vi "RT Main_V2 config.vi"   [LabVIEW 2015]
doc: "This template is for the Queued Message Handler design pattern.\n\nThe Event Handling Loop generates messages based on user interface actions.\n\nThe Message Handling Loop processes messages generated by the Event Handling Loop, or by other messages. The messages are string values, so new messages can be added easily to the Message Cases case structure in the Message Handling Loop. Each message cluster can also provide an optional value for Message Data, which is a variant that can be converted to whatever message-specific data is required."
uses:
  Globals/Global - All RT Loop Stop.vi
  Globals/Global - Monitoring Variables.vi
  Globals/Global - Configuration Options.vi
  Globals/Global - RT Stream Connections.vi
  support/Message Queue/Message Queue.lvlib
  <vilib>/nisyscfg/nisyscfg.lvlib
types:
  T1 = typedef "Acquisition and Logging Configuration_v1.ctl" = cluster{"Data Rate":T2, "Samples per Read":i32, "Number of Reads to Save":i32, "Data File Name":string, "TDMS Properties":T3[], "Number of Channels":i32, "Channel Scale Array":fxp<+,24,12>[], "Channel Names":string[], "Trigger - RMS Value":dbl, "Trigger - Channel":i32, "Trigger - Time (Minute)":i32, "Input Configuration Array":T4[]}
  T2 = typedef "nicrio_cRIO-9234_DataRatesRing2.ctl" = u8
  T3 = typedef "TDMS Properties.ctl" = cluster{"Name":string, "Value":string}
  T4 = typedef "nicrio_cRIO-9234_ConfigModeRing.ctl" = u8
  T5 = typedef "Message Queue.lvlib/All Real-Time Message Queues.ctl" = cluster{"Message Handler":refnum<queue>, "Acquisition and Logging":refnum<queue>}
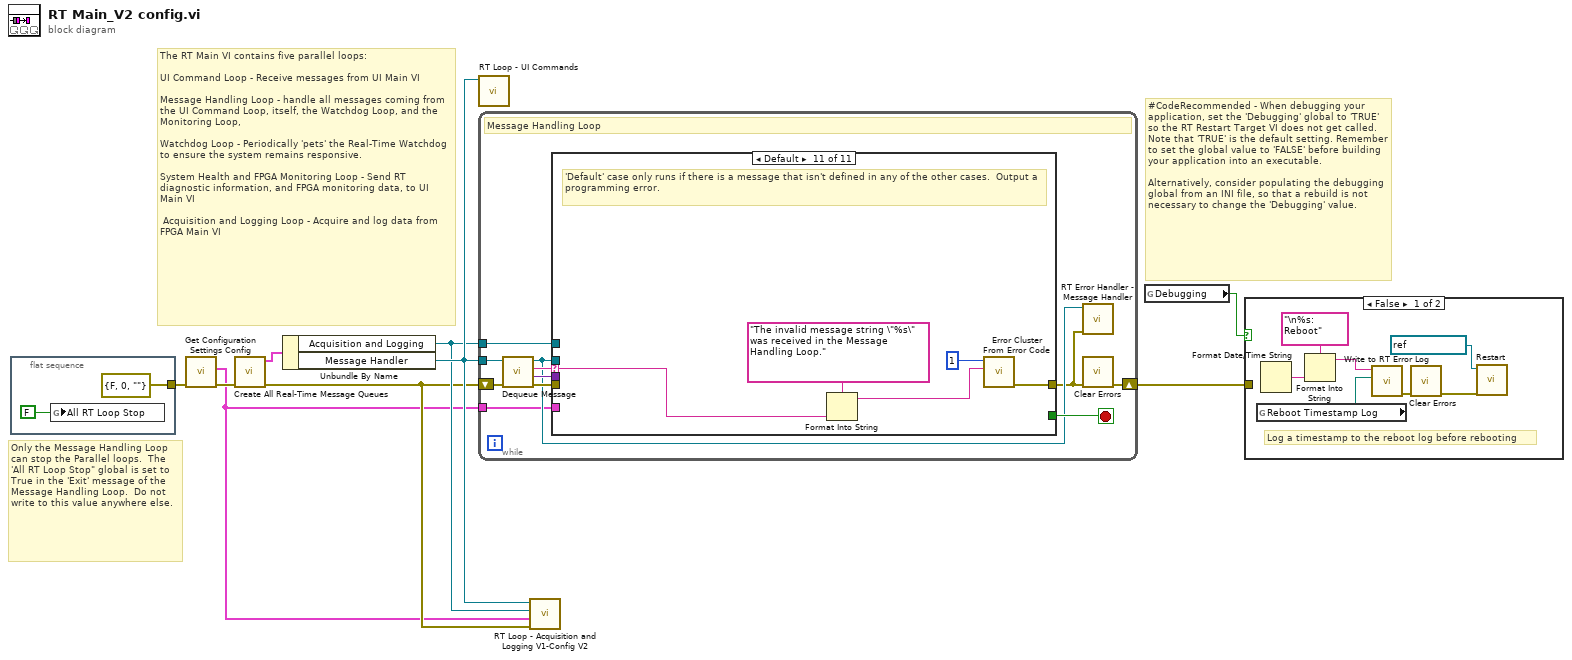
[diagram p0: block diagram]
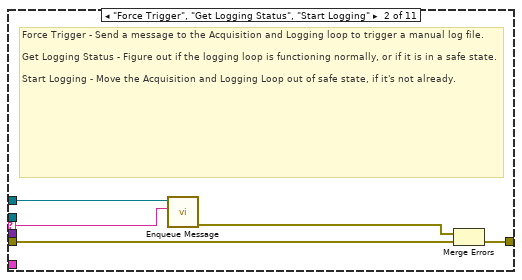
[diagram p4: hidden frame]
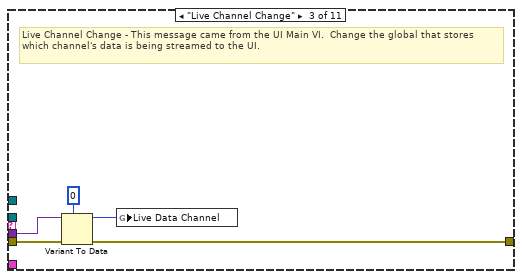
[diagram p5: hidden frame]
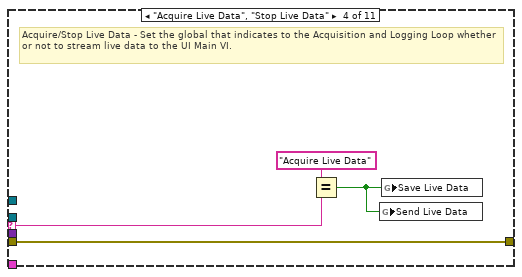
[diagram p6: hidden frame]
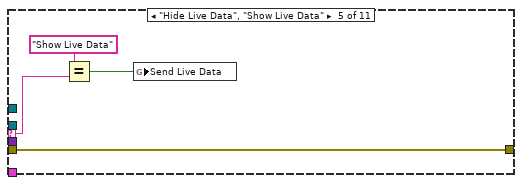
[diagram p7: hidden frame]
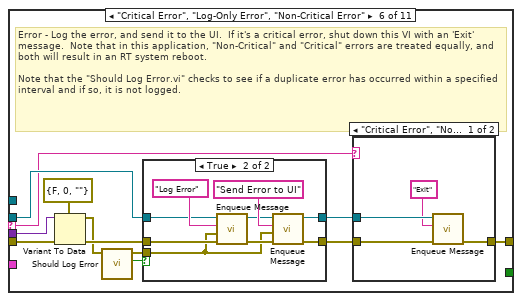
[diagram p8: hidden frame]
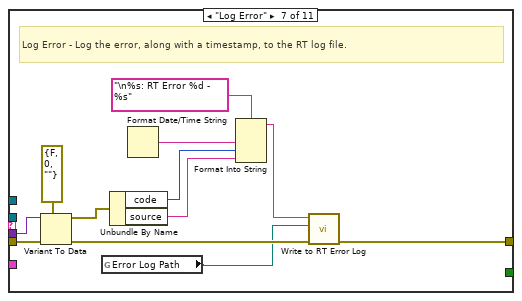
[diagram p11: hidden frame]
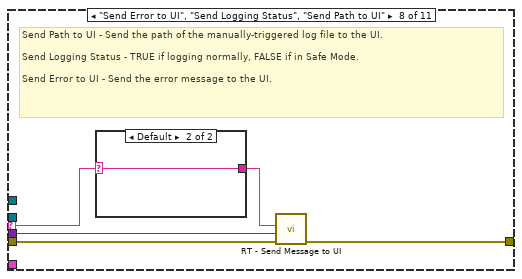
[diagram p12: hidden frame]
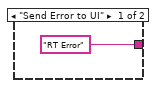
[diagram p13: hidden frame]
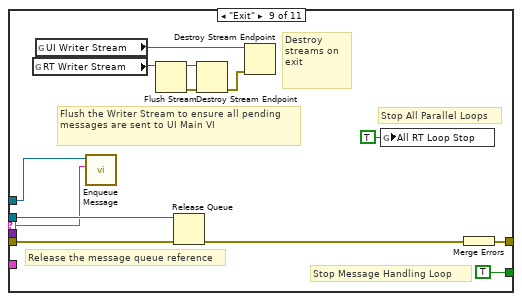
[diagram p14: hidden frame]
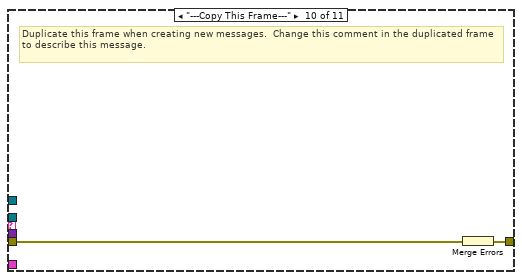
[diagram p15: hidden frame]
diagram:
  # "#CodeRecommended - When debugging your application, set the 'Debugging' global to 'TRUE' so the RT Restart Target VI does not get called.  Note that 'TRUE' is the default setting. Remember to set the global value to 'FALSE' before building your application into an executable.\n\nAlternatively, consider populating the debugging global from an INI file, so that a rebuild is not necessary to change the 'Debugging' value."
  # "The RT Main VI contains five parallel loops:\n\nUI Command Loop - Receive messages from UI Main VI\n\nMessage Handling Loop - handle all messages coming from the UI Command Loop, itself, the Watchdog Loop, and the Monitoring Loop, \n\nWatchdog Loop - Periodically 'pets' the Real-Time Watchdog to ensure the system remains responsive.\n\nSystem Health and FPGA Monitoring Loop - Send RT diagnostic information, and FPGA monitoring data, to UI Main VI\n\n Acquisition and Logging Loop - Acquire and log data from FPGA Main VI"
  # "Only the Message Handling Loop can stop the Parallel loops.  The 'All RT Loop Stop\" global is set to True in the 'Exit' message of the Message Handling Loop.  Do not write to this value anywhere else."
  n1 = flat-sequence {
    tunnel: [errorcluster {"status"=FALSE, "code"=0, "source"=""} ("error constant")] -> w9
    frame #0 {
      n2 = global write "Global - All RT Loop Stop.vi" "All RT Loop Stop"(FALSE) -> ()
    }
  }
  n3 = call "Get Configuration Settings Config.vi"("error in (no error)"=w9) -> ("error out"=w6:errorcluster, "Acquisition Data v1"=w1:T1)  [unwired: 9 in]
  n4 = call "Create All Real-Time Message Queues.vi"("error in (no error)"=w6) -> ("error out"=w2:errorcluster, "Message Queues out"=w5:T5)  [unwired: 9 in]
  n5 = Unbundle By Name(w5) -> ("Acquisition and Logging"=w3:refnum<queue>, "Message Handler"=w4:refnum<queue>)
  n6 = call "RT Loop - UI Commands.vi"("Message Queue"=w4) -> ()  [unwired: 11 in]
  n7 = while {
    tunnel: w4 -> [w17]
    shift-right: [w15] -> w8
    shift-left: w2 -> [w21]
    tunnel: w3 -> [w13]
    tunnel: w1 -> [w12]
    stop <- w22 stop-if-true
    # "Message Handling Loop"
    n8 = call "Dequeue Message.vi"("error in (no error)"=w21, "Message Queue"=w17) -> ("error out"=w20:errorcluster, "Message Data"=w18:variant, "Message"=w19:string, "dup Message Queue"=w16:refnum<queue>)  [unwired: 6 in]
    n9 = case "Message Cases" shown="Default" w19 {
      selector: w19 -> [_ w26 _ w36 w38 w47 _ w83 w91 _ w107]
      tunnel: w16 -> [_ _ _ _ _ w48 _ _ w101 _ _]
      tunnel: w20 -> [w23 w28 w33 w37 w41 w50 w81 w86 w97 w103 _]
      tunnel: [w23 w25 w32 w37 w41 w53 w72 w85 w98 w102 w105] -> w14
      tunnel: [_ _ _ _ _ _ _ _ TRUE _ _] -> w22
      tunnel: w18 -> [_ _ w31 _ _ w42 w80 w84 _ _ _]
      tunnel: w13 -> [_ w27 _ _ _ _ _ _ w92 _ _]
      tunnel: w12 -> [_ _ _ _ _ _ _ _ _ _ _]
      frame "Initialize" {
        # "Initialize - Currently a no-op for the RT Main VI"
      }
      frame "Force Trigger", "Get Logging Status", "Start Logging" {
        # "Force Trigger - Send a message to the Acquisition and Logging loop to trigger a manual log file.\n\nGet Logging Status - Figure out if the logging loop is functioning normally, or if it is in a safe state.\n\nStart Logging - Move the Acquisition and Logging Loop out of safe state, if it's not already."
        n10 = call "Enqueue Message.vi"("Message"=w26, "Message Queue"=w27) -> ("error out"=w24:errorcluster)  [unwired: 8 in, 1 out]
        n11 = Merge Errors(w24, w28) -> (w25:errorcluster)
      }
      frame "Live Channel Change" {
        # "Live Channel Change - This message came from the UI Main VI.  Change the global that stores which channel's data is being streamed to the UI."
        n12 = Variant To Data(error in=w33, type=u32 0, Variant=w31) -> (data=w29:u32, error out=w32:errorcluster)
        n13 = global write "Global - Monitoring Variables.vi" "Live Data Channel"(w29) -> ()
      }
      frame "Acquire Live Data", "Stop Live Data" {
        # "Acquire/Stop Live Data - Set the global that indicates to the Acquisition and Logging Loop whether or not to stream live data to the UI Main VI."
        n14 = Equal?(x="Acquire Live Data", y=w36) -> (x = y?=w34:bool)
        n15 = global write "Global - Monitoring Variables.vi" "Send Live Data"(w34) -> ()
        n16 = global write "Global - Monitoring Variables.vi" "Save Live Data"(w34) -> ()
      }
      frame "Hide Live Data", "Show Live Data" {
        n17 = Equal?(x="Show Live Data", y=w38) -> (x = y?=w39:bool)
        n18 = global write "Global - Monitoring Variables.vi" "Send Live Data"(w39) -> ()
      }
      frame "Critical Error", "Log-Only Error", "Non-Critical Error" {
        # "Error - Log the error, and send it to the UI.  If it's a critical error, shut down this VI with an 'Exit' message.  Note that in this application, \"Non-Critical\" and \"Critical\" errors are treated equally, and both will result in an RT system reboot.\n\nNote that the \"Should Log Error.vi\" checks to see if a duplicate error has occurred within a specified interval and if so, it is not logged."
        n19 = Variant To Data(error in=w50, type=errorcluster {"status"=FALSE, "code"=0, "source"=""} ("error out"), Variant=w42) -> (data=w45:errorcluster, error out=w51:errorcluster)
        n20 = call "Should Log Error.vi"("error to report"=w45) -> ("Should Log Error?"=w43:bool, "dup error to report"=w44:errorcluster)  [unwired: 9 in]
        n21 = case shown="True" w43 {
          tunnel: [w55 w62] -> w49
          tunnel: [w54 w61] -> w46
          tunnel: w48 -> [w54 w60]
          tunnel: w51 -> [w55 w57]
          tunnel: w44 -> [_ w56]
          frame False {
          }
          frame True {
            n22 = call "Enqueue Message.vi"("error in (no error)"=w57, "Message Data"=w56, "Message"="Log Error", "Message Queue"=w60) -> ("error out"=w58:errorcluster, "dup Message Queue"=w59:refnum<queue>)  [unwired: 6 in]
            n23 = call "Enqueue Message.vi"("error in (no error)"=w58, "Message Data"=w56, "Message"="Send Error to UI", "Message Queue"=w59) -> ("error out"=w62:errorcluster, "dup Message Queue"=w61:refnum<queue>)  [unwired: 6 in]
          }
        }
        n24 = case shown="\"Critical Error\", \"Non-Critical Error\"" w47 {
          tunnel: w49 -> [w68 w69]
          tunnel: w46 -> [w66 _]
          tunnel: [w67 w69] -> w53
          frame "Critical Error", "Non-Critical Error" {
            n25 = call "Enqueue Message.vi"("error in (no error)"=w68, "Message"="Exit", "Message Queue"=w66) -> ("error out"=w67:errorcluster)  [unwired: 7 in, 1 out]
          }
          frame Default {
          }
        }
      }
      frame "Log Error" {
        # "Log Error - Log the error, along with a timestamp, to the RT log file."
        n26 = Variant To Data(error in=w81, type=errorcluster {"status"=FALSE, "code"=0, "source"=""} ("error constant"), Variant=w80) -> (data=w75:errorcluster, error out=w78:errorcluster)
        n27 = global read "Global - Configuration Options.vi" "Error Log Path"() -> (w70:path)
        n28 = Unbundle By Name(w75) -> ("code"=w74:i32, "source"=w73:string)
        n29 = Format Date/Time String() -> (date/time string=w76:string)  [unwired: 3 in]
        n30 = Format Into String(format string="\n%s: RT Error %d - %s", w76, w74, w73) -> (resulting string=w71:string)  [unwired: 2 in, 1 out]
        n31 = call "Write to RT Error Log.vi"("error in (no error)"=w78, "Error Log Path"=w70, "Log Entry"=w71) -> ("error out"=w72:errorcluster)  [unwired: 8 in]
      }
      frame "Send Error to UI", "Send Logging Status", "Send Path to UI" {
        # "Send Path to UI - Send the path of the manually-triggered log file to the UI.\n\nSend Logging Status - TRUE if logging normally, FALSE if in Safe Mode.\n\nSend Error to UI - Send the error message to the UI."
        n32 = case shown="Default" w83 {
          selector: w83 -> [_ w88]
          tunnel: ["RT Error" ("Message") w88] -> w82
          frame "Send Error to UI" {
          }
          frame Default {
          }
        }
        n33 = call "RT - Send Message to UI.vi"("error in (no error)"=w86, "Message Data"=w84, "Message"=w82) -> ("error out"=w85:errorcluster)  [unwired: 8 in]
      }
      frame "Exit" {
        # "Flush the Writer Stream to ensure all pending messages are sent to UI Main VI"
        # "Destroy streams on exit"
        # "Stop Message Handling Loop"
        # "Stop All Parallel Loops"
        # "Release the message queue reference"
        n34 = global read "Global - RT Stream Connections.vi" "RT Writer Stream"() -> (w95:refnum<k21>)
        n35 = global read "Global - RT Stream Connections.vi" "UI Writer Stream"() -> (w94:refnum<k21>)
        n36 = call "Enqueue Message.vi"("Message"=w91, "Message Queue"=w92) -> ()  [unwired: 8 in, 2 out]
        n37 = Flush Stream(11:w95) -> (0:w89:errorcluster, 3:w90:refnum<k21>)  [unwired: 3 in, 1 out]
        n38 = Release Queue(queue=w101, error in (no error)=w97) -> (error out=w99:errorcluster)  [unwired: 1 in, 2 out]
        n39 = Destroy Stream Endpoint(8:w89, 11:w90) -> (0:w93:errorcluster)
        n40 = Destroy Stream Endpoint(8:w93, 11:w94) -> ()  [unwired: 1 out]
        n41 = global write "Global - All RT Loop Stop.vi" "All RT Loop Stop"(TRUE ("Stop Monitoring Loops")) -> ()
        n42 = Merge Errors(w99) -> (w98:errorcluster)
      }
      frame "---Copy This Frame---" {
        # "Duplicate this frame when creating new messages.  Change this comment in the duplicated frame to describe this message."
        n43 = Merge Errors(w103) -> (w102:errorcluster)
      }
      frame Default {
        # "'Default' case only runs if there is a message that isn't defined in any of the other cases.  Output a programming error."
        n44 = Format Into String(format string="The invalid message string \"%s\" was received in the Message Handling Loop." ("Unknown Message Error Text"), w107) -> (resulting string=w104:string)  [unwired: 2 in, 1 out]
        n45 = call <vilib>:"Error Cluster From Error Code.vi"("error message (\"\")"=w104, "error code (0)"=1) -> ("error out"=w105:errorcluster)  [unwired: 7 in]
      }
    }
    n46 = call "RT Error Handler - Message Handler.vi"("error in (no error)"=w14, "Message Queue"=w16) -> ()  [unwired: 9 in, 1 out]
    n47 = call <vilib>:"Clear Errors.vi"("error in (no error)"=w14) -> ("error out"=w15:errorcluster)  [unwired: 5 in, 1 out]
  }
  n48 = call "RT Loop - Acquisition and Logging V1-Config V2.vi"("error in (no error)"=w2, "Acquisition Data v1"=w1, "Acquisition and Logging Queue"=w3, "Message Queue"=w4) -> ()  [unwired: 8 in]
  n49 = global read "Global - Configuration Options.vi" "Debugging"() -> (w7:bool)
  n50 = case shown="False" w7 {
    tunnel: w8 -> [_ _]
    frame False {
      # "Log a timestamp to the reboot log before rebooting"
      n51 = global read "Global - Configuration Options.vi" "Reboot Timestamp Log"() -> (w111:path)
      n52 = Format Date/Time String() -> (date/time string=w113:string)  [unwired: 3 in]
      n53 = Format Into String(format string="\n%s: Reboot", w113) -> (resulting string=w112:string)  [unwired: 2 in, 1 out]
      n54 = call "Write to RT Error Log.vi"("Error Log Path"=w111, "Log Entry"=w112) -> ("error out"=w115:errorcluster)  [unwired: 9 in]
      n55 = call <vilib>:"Clear Errors.vi"("error in (no error)"=w115) -> ("error out"=w110:errorcluster)  [unwired: 5 in, 1 out]
      n56 = call <vilib>:"Restart.vi"("error in (no error)"=w110, "Session in"=refnum<k21> "localhost" ("session in")) -> ()  [unwired: 7 in, 3 out]
    }
    frame True {
    }
  }
